vi "Create Donut Plot.vi"(6 "target image filepath":path, 7 "plot colors":u32[](array[colorbox]), 8 "error in (no error)":errorcluster, 9 "labels":T1, 10 "datasets":dbl[](array[numeric])) -> (0 "error out":errorcluster, 2 "donut plot":picture)   [LabVIEW 2019, in "Python Visualizations.lvlib"]
uses:
  Python Visualizations.lvlib
  pieplot_labels.ctl
  <vilib>/Utility/sysdir.llb/System Directory Type.ctl
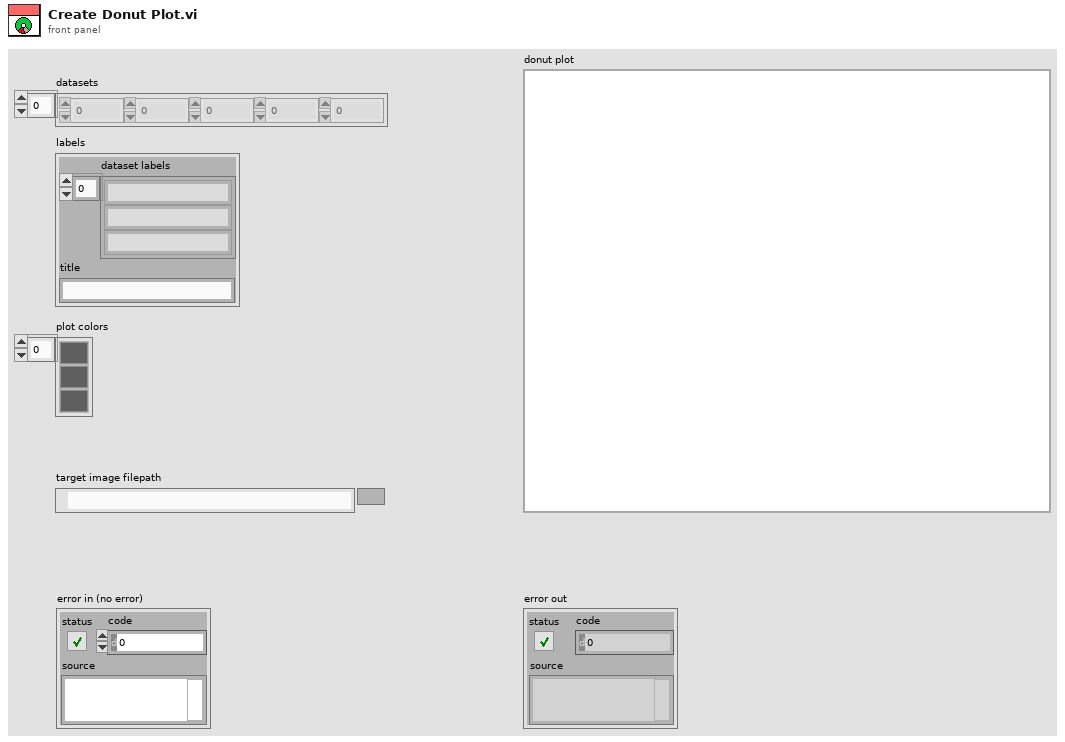
[diagram p1: front panel]
types:
  T1 = typedef "Python Visualizations.lvlib/pieplot_labels.ctl" = cluster{"dataset labels":string[], "title":string}
  T2 = typedef "System Directory Type.ctl" = i32
  T3 = typedef "imagedata.ctl" = cluster{"image type":i32, "image depth":i32, "image":u8[], "mask":u8[], "colors":u32[], "Rectangle":cluster{"left":i16, "top":i16, "right":i16, "bottom":i16}}
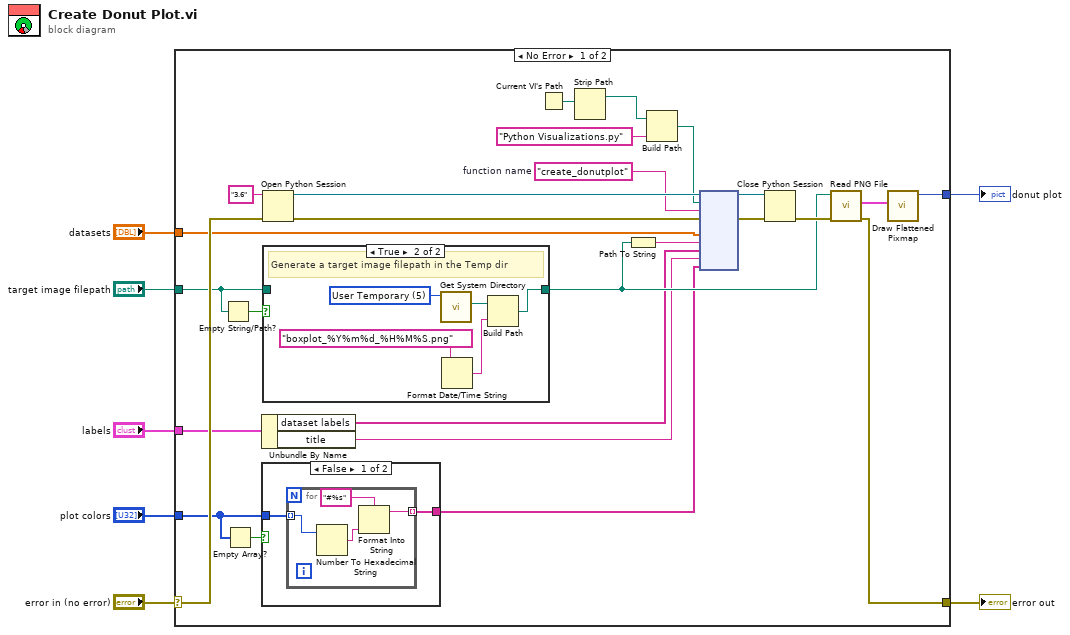
[diagram p0: block diagram]
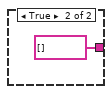
[diagram p2: hidden frame]
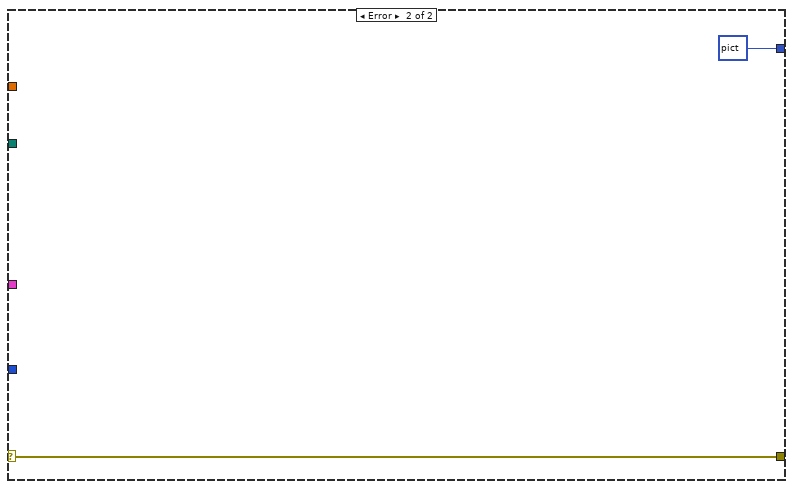
[diagram p4: hidden frame]
diagram:
  n1 = case shown="No Error" "error in (no error)" {
    selector: "error in (no error)" -> [w22 w48]
    tunnel: [w24 picture data[5B] ("new picture")] -> w7
    tunnel: [w21 w48] -> w5
    tunnel: "target image filepath" -> [w16 _]
    tunnel: "datasets" -> [w14 _]
    tunnel: "labels" -> [w13 _]
    tunnel: "plot colors" -> [w9 _]
    frame No Error {
      w28 = "create_donutplot"  # function name
      n2 = Empty String/Path?(string/path=w16) -> (empty?=w17:bool)
      n3 = Empty Array?(array=w9) -> (empty?=w8:bool)
      n4 = Unbundle By Name(w13) -> ("dataset labels"=w12:string[], "title"=w11:string)
      n5 = case shown="False" w8 {
        tunnel: [w35 string[] []] -> w10
        tunnel: w9 -> [w34 _]
        frame False {
          n6 = for {
            tunnel: w34 -> [w39] mode=indexing
            tunnel: [w36] -> w35 mode=indexing
            n7 = Number To Hexadecimal String(2:w39) -> (0:w38:string)  [unwired: 1 in]
            n8 = Format Into String(format string="#%s", w38) -> (resulting string=w36:string)  [unwired: 2 in, 1 out]
          }
        }
        frame True {
        }
      }
      n9 = Open Python Session(python version="3.6" ("Python version"), 3:w22) -> (session out=w33:refnum<k35>, error out=w31:errorcluster)  [unwired: 1 in]
      n10 = case shown="True" w17 {
        tunnel: w16 -> [w41 _]
        tunnel: [w41 w42] -> w15
        frame False {
          # "Caller has specified a target image filepath"
        }
        frame True {
          w46 = T2 5 items=["User Home"=0, "User Desktop"=1, "User Documents"=2, "User Application Data"=3, "User Preferences"=4, "User Temporary"=5, "Public Documents"=6, "Public Application Data"=7, "Public Preferences"=8, "Public Cache"=13, "System Core Libraries"=9, "System Installed Libraries"=10, "Application Files"=11, "Boot Volume Root"=12] ("system directory type")
          # "Generate a target image filepath in the Temp dir"
          n11 = call <vilib>:"Get System Directory.vi"("system directory type"=w46) -> ("system directory"=w45:path)  [unwired: 10 in]
          n12 = Format Date/Time String(time format string (%c)="boxplot_%Y%m%d_%H%M%S.png") -> (date/time string=w43:string)  [unwired: 2 in]
          n13 = Build Path(base path=w45, name or relative path=w43) -> (appended path=w42:path)
        }
      }
      n14 = Current VI's Path() -> (path=w19:path)
      n15 = Strip Path(path=w19) -> (stripped path=w18:path)  [unwired: 1 out]
      n16 = Path To String(path=w15) -> (string=w32:string)
      n17 = Build Path(base path=w18, name or relative path="Python Visualizations.py") -> (appended path=w29:path)
      n18 = node(w33, w29, w28, w31, w14, w32, w12, w11, w10) -> (w27:refnum<k35>, w26:errorcluster)  [unwired: 7 in, 2 out]
      n19 = Close Python Session(session in=w27, error in=w26) -> (11:w23:errorcluster)
      n20 = call <vilib>:"Read PNG File.vi"("error in (no error)"=w23, "path to PNG file"=w15) -> ("error out"=w21:errorcluster, "image data"=w25:T3)  [unwired: 7 in, 1 out]
      n21 = call <vilib>:"Draw Flattened Pixmap.vi"("image data"=w25) -> ("new picture"=w24:picture)  [unwired: 8 in]
    }
    frame Error {
    }
  }
  "error out" <- w5
  "donut plot" <- w7
